vi "test Swap Data.vi"(8 "error in (no error)":errorcluster, 11 "TestCase in":refnum<class "Data Manipulation Tests.lvclass">) -> (0 "error out":errorcluster, 3 "TestCase out":refnum<class "Data Manipulation Tests.lvclass">)   [LabVIEW 2017, in "Pointer Tests.lvlib" / "Data Manipulation Tests.lvclass"]
uses:
  Data Manipulation Tests.lvclass
  Source/Classes/Pointer/Pointer.lvclass/Pointer.ctl
  Source/Classes/Pointer/Public/New/New (4B).vi
  Source/Classes/Pointer/Public/Write/Write (1D I32).vi
  Source/Classes/Pointer/Public/Read/Read (1D I32).vi
  Source/Classes/Pointer/Private/Allocate.vi
  Source/Classes/Pointer/Public/Write (No Check)/Write (No Check 1D I32).vi
  Source/Classes/Pointer/Protected/Parameter Checking/Check Null Pointer.vi
  Source/Classes/Pointer/Protected/Parameter Checking/Check Subset (Power of 2).vi
  Source/Classes/Pointer/API/Accessors/Get Size.vi
  Source/Classes/Pointer/Protected/Errors.vi
  Source/Classes/Pointer/Protected/Error VIs/Size Mismatch.vi
  Source/Classes/Pointer/Public/Swap (No Check).vi
  Source/Classes/Pointer/Public/Read (No Check)/Read (No Check 1D I32).vi
  Source/Classes/Pointer/Private/Deallocate.vi
  Source/Classes/Pointer/API/Accessors/Set Address.vi
  Source/Classes/Pointer/API/Accessors/Set Size.vi
  Source/Classes/Pointer/Private/Set Internal.vi
  Source/Classes/Pointer/API/Accessors/Get Address.vi
  Source/Classes/Pointer/Protected/Error VIs/Null Pointer.vi
  Source/Classes/Pointer/Protected/Error VIs/Out of Bounds.vi
  Source/Classes/Pointer/Private/Count to Size.vi
  Source/Classes/Pointer/Protected/Error Building/Create Error.vi
  Source/VIs/Write String into Source.vi
  Source/VIs/Write Number into Source.vi
  Source/VIs/VIs for Poly/Write U64 into Source.vi
  Source/Classes/Pointer/Protected/Get Internal.vi
  Source/Classes/Pointer/Protected/Error VIs/Zone.vi
  Source/Classes/Pointer/Protected/Error Building/Write Pointer Size.vi
  Source/Constants/Constants.vi
  Source/Constants/Library Name.vi
  Source/Classes/Pointer/Protected/Error Building/Get Error Info.vi
  Source/VIs/Create Error Cluster.vi
  Source/VIs/VIs for Poly/Create Error Cluster (256B).vi
  Source/VIs/Set Error Status.vi
  Source/VIs/Set Error Code.vi
  Source/VIs/Set Error Source.vi
  Source/Classes/Pointer/Pointer.lvclass
  <vilib>/addons/_JKI Toolkits/VI Tester/TestCase.llb/TestCase.lvclass
  C:/Program Files (x86)/National Instruments/LabVIEW 2017/vi.lib/addons/_JKI Toolkits/VI Tester/TestCase.llb/TestCase.lvclass
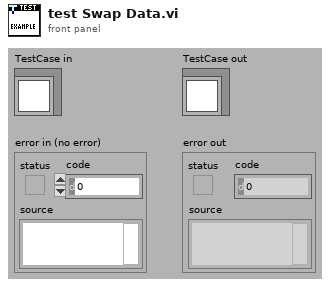
[diagram p1: front panel]
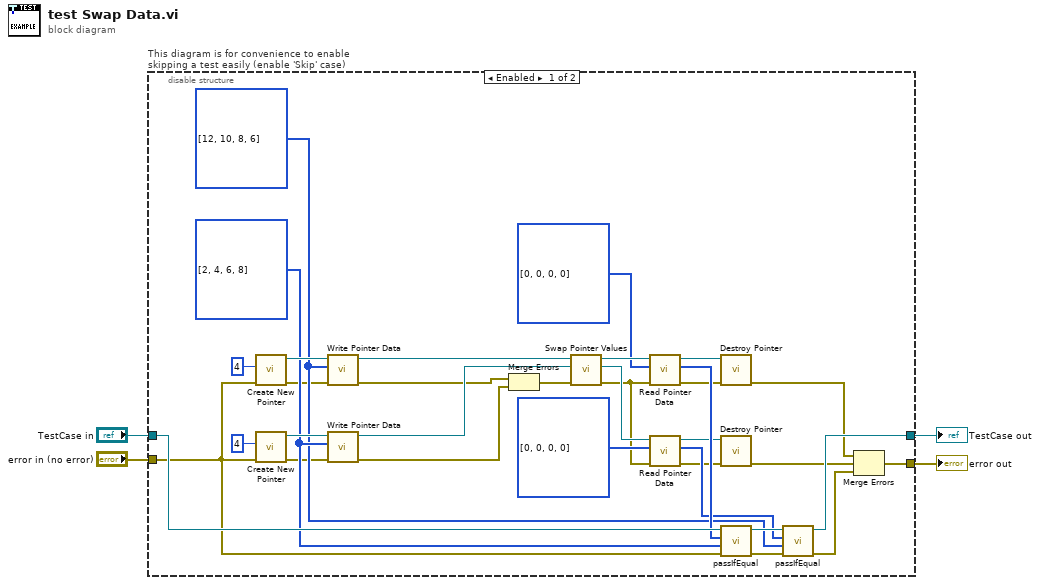
[diagram p0: block diagram]
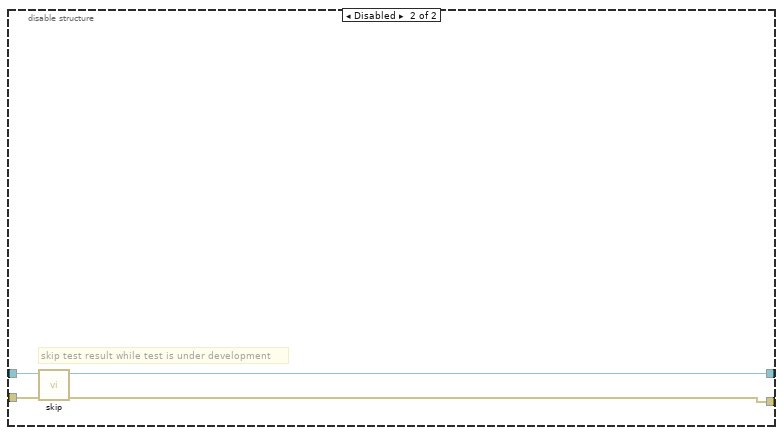
[diagram p2: hidden frame]
diagram:
  n1 = disable-structure "This diagram is for convenience to enable skipping a test easily (enable 'Skip' case)" shown="Enabled" {
    disable-tunnel: "TestCase in" -> [w27 w41]
    disable-tunnel: [w20 w39] -> w1
    disable-tunnel: [w11 w40] -> w3
    disable-tunnel: "error in (no error)" -> [w12 w38]
    frame Enabled {
      w25 = i32[] [2, 4, 6, 8] ("buffer in")
      w21 = i32[] [12, 10, 8, 6] ("buffer in")
      n2 = call-poly "Create New Pointer.vi"("error in (no error)"=w12, "count (1)"=u64 4) -> ("error out"=w14:errorcluster, "Pointer"=w35:refnum<class "Pointer.lvclass">)  [unwired: 8 in]
      n3 = call-poly "Create New Pointer.vi"("error in (no error)"=w12, "count (1)"=u64 4) -> ("error out"=w18:errorcluster, "Pointer"=w34:refnum<class "Pointer.lvclass">)  [unwired: 8 in]
      n4 = call-poly "Write Pointer Data.vi"("error in (no error)"=w14, "buffer in"=w21, "Pointer in"=w35) -> ("error out"=w15:errorcluster, "Pointer out"=w33:refnum<class "Pointer.lvclass">)  [unwired: 5 in, 2 out]
      n5 = call-poly "Write Pointer Data.vi"("error in (no error)"=w18, "buffer in"=w25, "Pointer in"=w34) -> ("error out"=w17:errorcluster, "Pointer out"=w32:refnum<class "Pointer.lvclass">)  [unwired: 5 in, 2 out]
      n6 = Merge Errors(w15, w17) -> (w16:errorcluster)
      n7 = call "Swap Pointer Values.vi"("error in (no error)"=w16, "Pointer b"=w32, "Pointer a"=w33) -> ("error out"=w13:errorcluster, "Pointer b"=w30:refnum<class "Pointer.lvclass">, "Pointer a"=w31:refnum<class "Pointer.lvclass">)  [unwired: 6 in]
      n8 = call-poly "Read Pointer Data.vi"("error in (no error)"=w13, "buffer in"=i32[] [0, 0, 0, 0], "Pointer in"=w31) -> ("error out"=w9:errorcluster, "buffer out"=w26:i32[], "Pointer out"=w7:refnum<class "Pointer.lvclass">)  [unwired: 5 in, 1 out]
      n9 = call-poly "Read Pointer Data.vi"("error in (no error)"=w13, "buffer in"=i32[] [0, 0, 0, 0], "Pointer in"=w30) -> ("error out"=w10:errorcluster, "buffer out"=w22:i32[], "Pointer out"=w8:refnum<class "Pointer.lvclass">)  [unwired: 5 in, 1 out]
      n10 = call "Destroy Pointer.vi"("error in (no error)"=w9, "Pointer in"=w7) -> ("error out"=w6:errorcluster)  [unwired: 8 in, 1 out]
      n11 = call "Destroy Pointer.vi"("error in (no error)"=w10, "Pointer in"=w8) -> ("error out"=w5:errorcluster)  [unwired: 8 in, 1 out]
      n12 = call-dynamic "passIfEqual.vi"("error in (no error)"=w12, "y"=w25, "x"=w26, "TestCase in"=w27) -> ("error out"=w24:errorcluster, "TestCase out"=w23:refnum<class "Data Manipulation Tests.lvclass">)  [unwired: 6 in]
      n13 = call-dynamic "passIfEqual.vi"("error in (no error)"=w24, "y"=w21, "x"=w22, "TestCase in"=w23) -> ("error out"=w19:errorcluster, "TestCase out"=w20:refnum<class "Data Manipulation Tests.lvclass">)  [unwired: 6 in]
      n14 = Merge Errors(w6, w5, w19) -> (w11:errorcluster)
    }
    frame Disabled {
      # "skip test result while test is under development"
      n15 = call <vilib>:"skip.vi"("error in (no error)"=w38, "TestCase in"=w41) -> ("error out"=w40:errorcluster, "TestCase out"=w39:refnum<class "Data Manipulation Tests.lvclass">)  [unwired: 8 in]
    }
  }
  "error out" <- w3
  "TestCase out" <- w1
